vi "Restart GUI.vi"(8 "error in (no error)":errorcluster, 11 "Wait (seconds)":u32=10) -> (3 "Abort out":bool)   [LabVIEW 2014, in "NIAnalysis.lvlib"]
uses:
  NIAnalysis.lvlib
panel:
  in  "Abort":bool
  in  "Restart":bool
  out "Message":string
  out "Code":i32
  out "Error":bool
  out "Time to Restart":u32
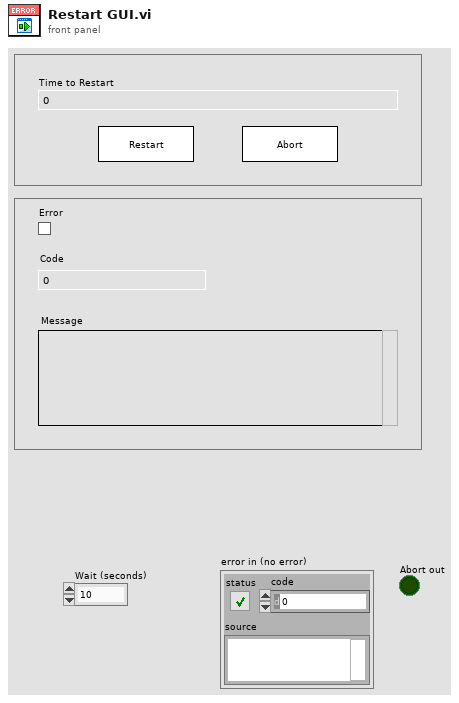
[diagram p1: front panel]
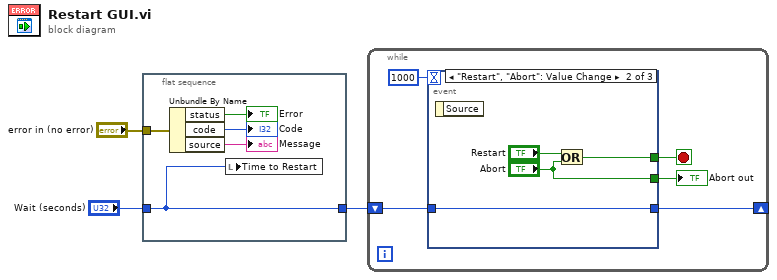
[diagram p0: block diagram]
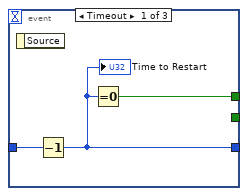
[diagram p2: hidden frame]
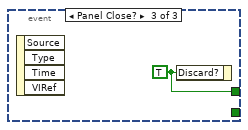
[diagram p3: hidden frame]
diagram:
  n1 = flat-sequence {
    tunnel: "error in (no error)" -> [w5]
    tunnel: "Wait (seconds)" -> [w4]
    tunnel: [w4] -> w1
    frame #0 {
      n2 = Unbundle By Name(w5) -> ("status"=→"Error":bool, "code"=→"Code":i32, "source"=→"Message":string)
      n3 = local write "Time to Restart"(w4) -> ()
    }
  }
  n4 = while {
    shift-right: [w11] -> _
    shift-left: w1 -> [w12]
    stop <- w10 stop-if-true
    n5 = event shown="[1] \"Restart\", \"Abort\": Value Change" {
      selector: _ -> [_ _ _]
      dyn-events: _ -> [_ _ _]
      timeout: 1000 -> [_ _ _]
      tunnel: w12 -> [w16 w20 _]
      tunnel: [w15 w20 _] -> w11
      tunnel: [w14 w18 w21] -> w10
      tunnel: [_ "Abort" _] -> w9
      event Timeout {
        n6 = event-data() -> ()  [unwired: 1 in, 1 out]
        n7 = Decrement(x=w16) -> (x-1=w15:u32)
        "Time to Restart" <- w15
        n8 = Equal To 0?(x=w15) -> (x = 0?=w14:bool)
      }
      event "Restart", "Abort": Value Change {
        n9 = event-data() -> ()  [unwired: 1 in, 1 out]
        n10 = Or(x="Restart", y="Abort") -> (x .or. y?=w18:bool)
      }
      event Panel Close? {
        w21 = TRUE ("Discard?")
        n11 = event-data() -> ()  [unwired: 1 in, 4 out]
        n12 = event-data("Discard?"=w21) -> ()  [unwired: 1 in, 1 out]
      }
    }
    "Abort out" <- w9
  }
